vi "73XX Motion Controller RT Driver VI.vi"(7 "Operation":T1, 11 "Device Reference in":T2 format="%.0x") -> (0 "Error Code":i32)   [LabVIEW 2010, in "73XX Motion Controller Custom Device.lvlib"]
uses:
  73XX Motion Controller Custom Device.lvlib
  <vilib>/NI VeriStand/Custom Device API/Custom Device Item Ref.ctl
  <vilib>/NI VeriStand/Custom Device API/Hardware Interface Driver VI Operation.ctl
  <vilib>/NI VeriStand/Custom Device API/Data Reference.ctl
  <vilib>/NI VeriStand/Custom Device API/Custom Device Channel Type.ctl
  <vilib>/NI VeriStand/Custom Device API/Data Access Type.ctl
  <vilib>/NI VeriStand/Custom Device API/Get Item Property (U16).vi
  <vilib>/Motion/FlexMotion/FunctionsVIs/StartStopMotion.llb/Start Motion (8 axes).flx
  <vilib>/Motion/FlexMotion/FunctionsVIs/StartStopMotion.llb/Stop Motion (8 axes).flx
  <vilib>/NI Veristand/Custom Device API/Custom Device API.lvlib
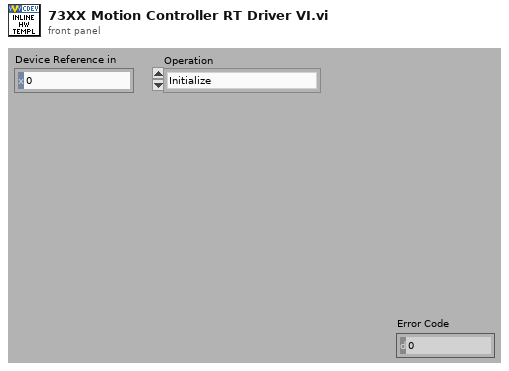
[diagram p1: front panel]
types:
  T1 = typedef "Custom Device API.lvlib/Hardware Interface Driver VI Operation.ctl" = enum16{"Initialize", "Start", "Read Data from HW", "Write Data to HW", "Close"}
  T2 = typedef "Custom Device API.lvlib/Custom Device Item Ref.ctl" = u64
  T3 = typedef "Custom Device API.lvlib/Data Reference.ctl" = i32
  T4 = cluster{"Device Error":errorcluster, "Current Position":i32, "Board ID":u16, "Axis":u16, "Velocity":u16, "Velocity Ref":T3, "Current Position Ref":T3, "Current Velcoity":i32, "Target Position":i32, "Target Position Ref":T3, "Current Velocity Ref":T3, "Reset Position? Ref":T3, "Reset Position?":T3, "Operation Mode":T3}
  T5 = typedef "Custom Device API.lvlib/Custom Device Channel Type.ctl" = enum16{"Input", "Output"}
  T6 = enum16{"Absolute Position", "Relative Position", "Velocity", "Relative to Cap Pos", "Modulus Position", "Absolute Contouring", "Relative Contouring"}
  T7 = typedef "Custom Device API.lvlib/Data Access Type.ctl" = enum16{"Read", "Write"}
  T8 = typedef "Bd Id Out" = u8
  T9 = typedef "Resource Out (Enum).flx" = u16
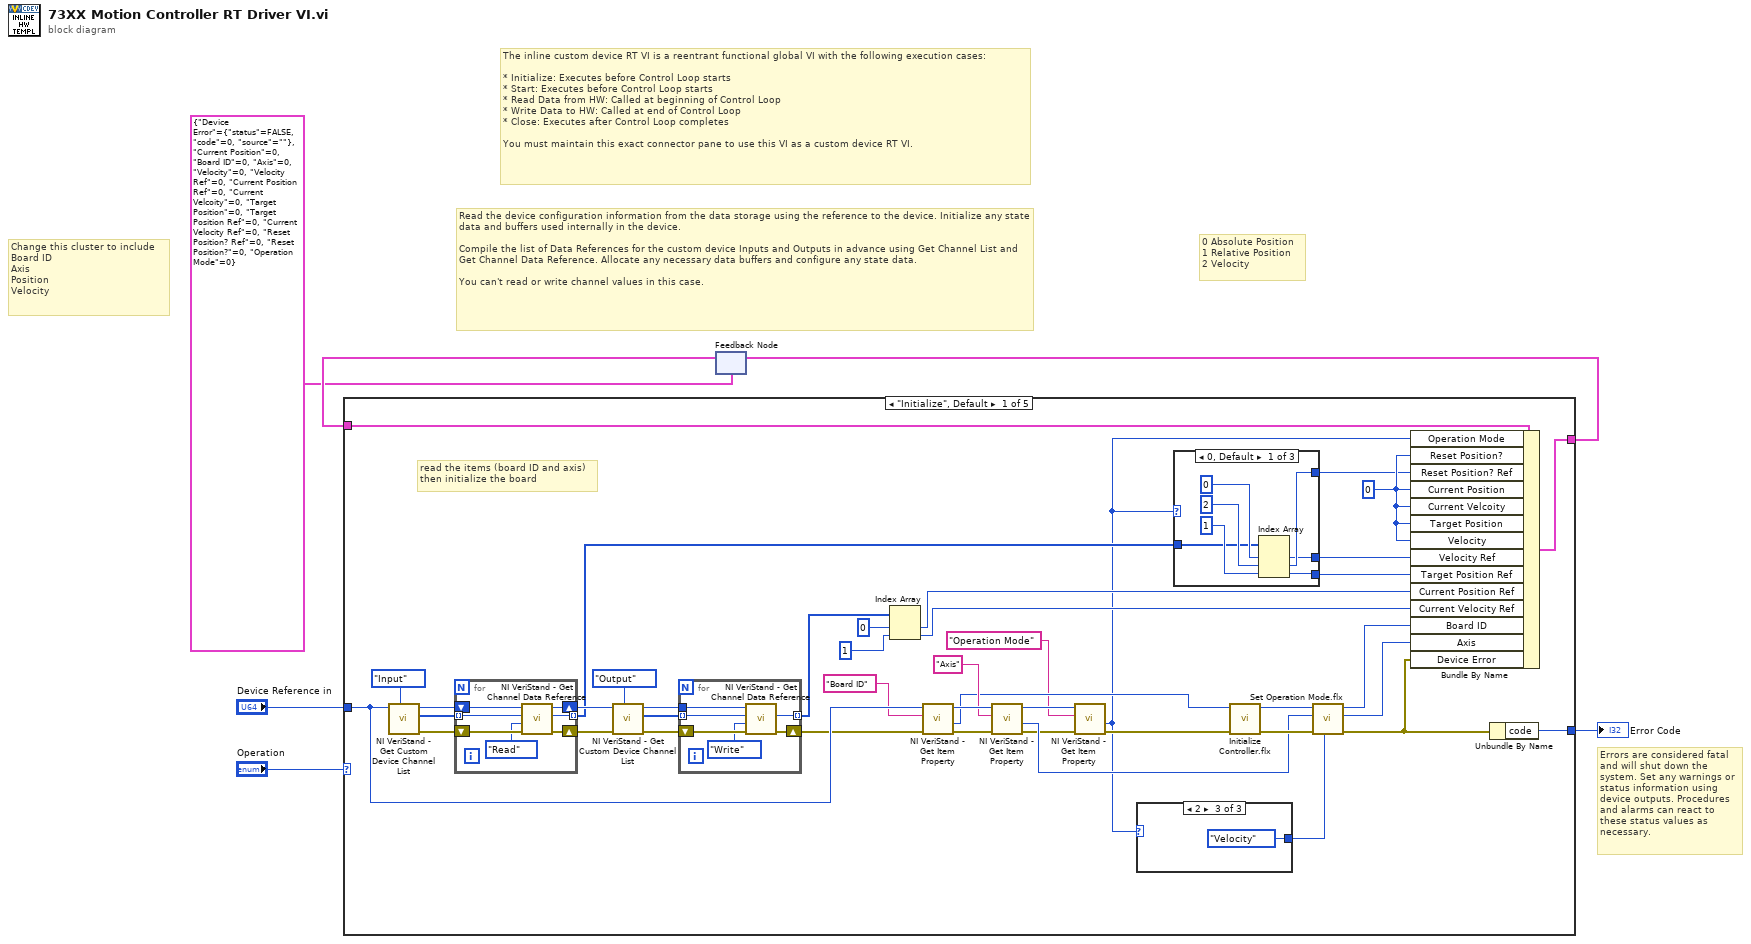
[diagram p0: block diagram]
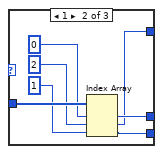
[diagram p2: hidden frame]
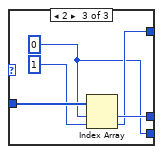
[diagram p3: hidden frame]
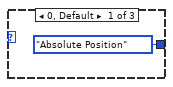
[diagram p4: hidden frame]
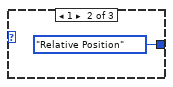
[diagram p5: hidden frame]
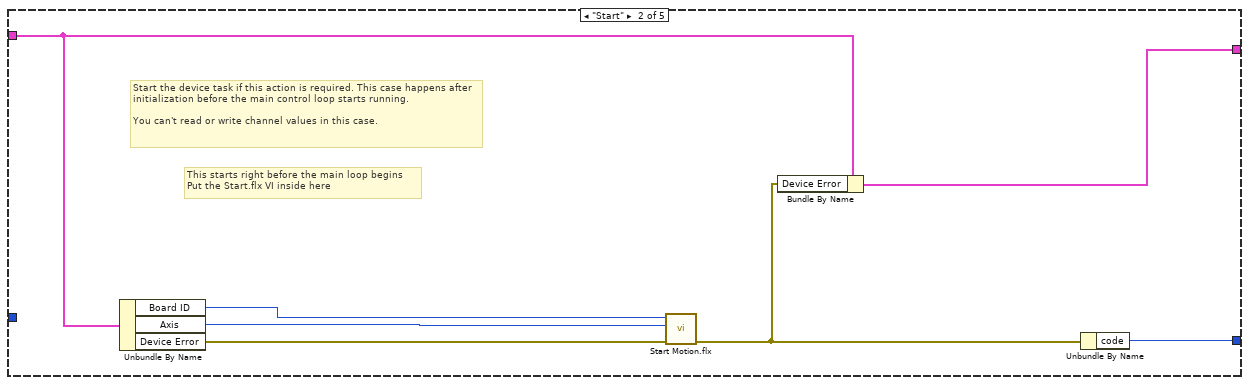
[diagram p6: hidden frame]
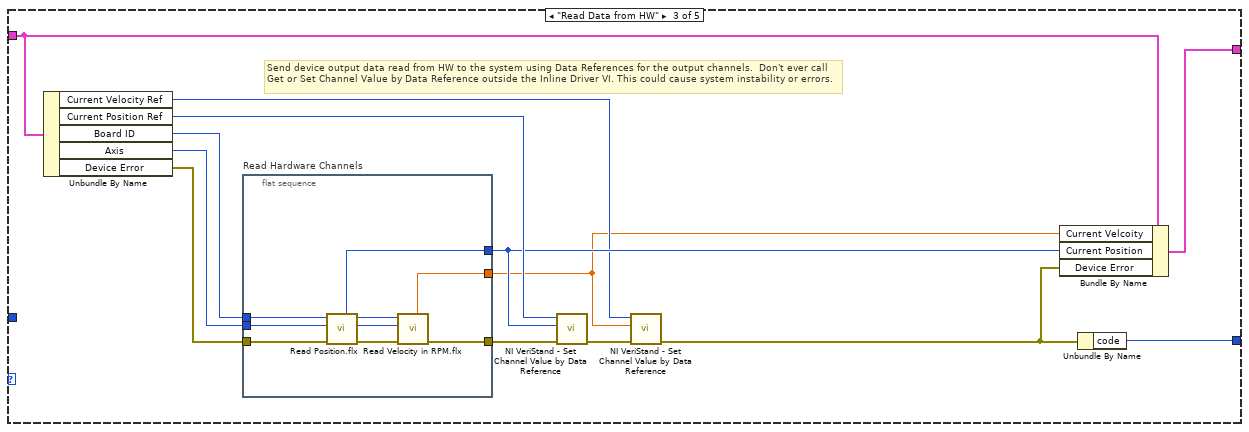
[diagram p7: hidden frame]
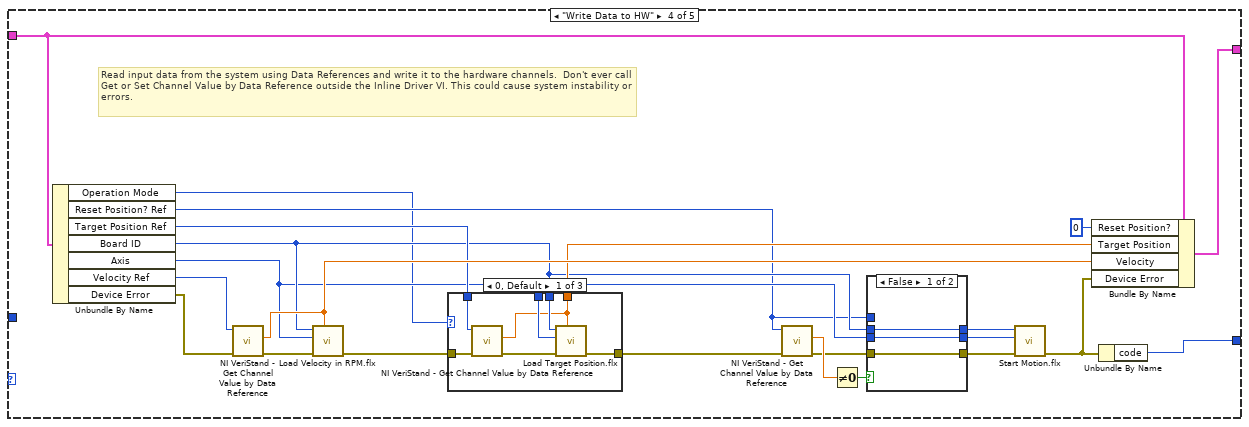
[diagram p8: hidden frame]
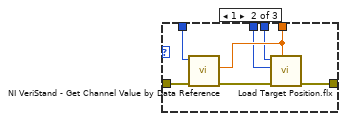
[diagram p9: hidden frame]
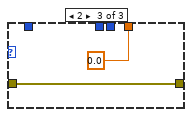
[diagram p10: hidden frame]
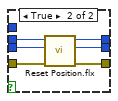
[diagram p11: hidden frame]
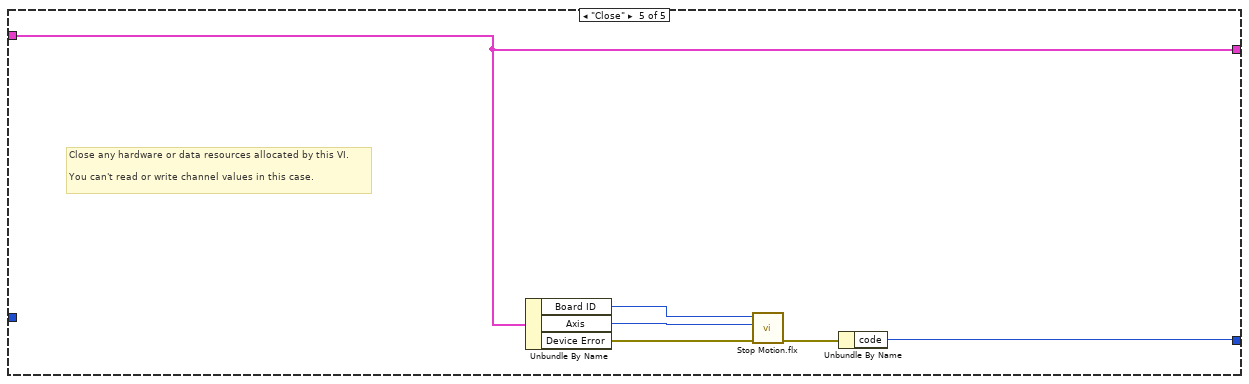
[diagram p12: hidden frame]
diagram:
  # "0 Absolute Position\n1 Relative Position\n2 Velocity"
  # "Change this cluster to include\nBoard ID\nAxis\nPosition\nVelocity"
  # "Read the device configuration information from the data storage using the reference to the device. Initialize any state data and buffers used internally in the device.\n\nCompile the list of Data References for the custom device Inputs and Outputs in advance using Get Channel List and Get Channel Data Reference. Allocate any necessary data buffers and configure any state data.\n\nYou can't read or write channel values in this case."
  # "Errors are considered fatal and will shut down the system. Set any warnings or status information using device outputs. Procedures and alarms can react to these status values as necessary."
  # "The inline custom device RT VI is a reentrant functional global VI with the following execution cases:\n\n* Initialize: Executes before Control Loop starts\n* Start: Executes before Control Loop starts\n* Read Data from HW: Called at beginning of Control Loop\n* Write Data to HW: Called at end of Control Loop\n* Close: Executes after Control Loop completes\n\nYou must maintain this exact connector pane to use this VI as a custom device RT VI."
  n1 = feedback #1(T4 {"Device Error"={"status"=FALSE, "code"=0, "source"=""}, "Current Position"=0, "Board ID"=0, "Axis"=0, "Velocity"=0, "Velocity Ref"=0, "Current Position Ref"=0, "Current Velcoity"=0, "Target Position"=0, "Target Position Ref"=0, "Current Velocity Ref"=0, "Reset Position? Ref"=0, "Reset Position?"=0, "Operation Mode"=0} ("cluster")) -> (w4:T4)
  n2 = case shown="\"Initialize\", Default" "Operation" {
    tunnel: [w27 w89 w99 w134 w166] -> w5
    tunnel: w4 -> [w28 w90 w100 w135 w166]
    tunnel: "Device Reference in" -> [w35 _ _ _ _]
    tunnel: [w47 w87 w102 w132 w161] -> w2
    frame "Initialize", Default {
      w14 = 0 ("element")
      # "read the items (board ID and axis)\nthen initialize the board"
      n3 = call <vilib>:"NI VeriStand - Get Custom Device Channel List.vi"("Channel Type"=Custom_Device_Channel_Type."Input", "Device Ref in"=w35) -> ("error out"=w45:errorcluster, "Specified Channel Ref List"=w44:T2[], "Device Ref out"=w46:T2)  [unwired: 1 in, 6 out]
      n4 = for {
        shift-right: [w78] -> w40
        shift-left: w46 -> [w82]
        tunnel: w44 -> [w81] mode=indexing
        shift-right: [w79] -> w39
        shift-left: w45 -> [w83]
        tunnel: [w77] -> w30 mode=indexing
        n5 = call <vilib>:"NI VeriStand - Get Channel Data Reference.vi"("error in (no error)"=w83, "Access"=Data_Access_Type."Read", "Channel Ref in"=w81, "Device Ref in"=w82) -> ("error out"=w79:errorcluster, "Channel Data Reference"=w77:T3, "Device Ref out"=w78:T2)  [unwired: 5 out]
      }
      n6 = call <vilib>:"NI VeriStand - Get Custom Device Channel List.vi"("Channel Type"=Custom_Device_Channel_Type."Output", "error in (no error)"=w39, "Device Ref in"=w40) -> ("error out"=w43:errorcluster, "Specified Channel Ref List"=w38:T2[], "Device Ref out"=w42:T2)  [unwired: 6 out]
      n7 = for {
        tunnel: w38 -> [w74] mode=indexing
        shift-right: [w72] -> w32
        shift-left: w43 -> [w76]
        tunnel: [w71] -> w31 mode=indexing
        tunnel: w42 -> [w75]
        n8 = call <vilib>:"NI VeriStand - Get Channel Data Reference.vi"("error in (no error)"=w76, "Access"=Data_Access_Type."Write", "Channel Ref in"=w74, "Device Ref in"=w75) -> ("error out"=w72:errorcluster, "Channel Data Reference"=w71:T3)  [unwired: 6 out]
      }
      n9 = Index Array(array=w31, index #1=0 ("index"), index #2=1 ("index")) -> (element #1=w25:T3, element #2=w23:T3)
      n10 = call-poly <vilib>:"NI VeriStand - Get Item Property.vi"("error in (no error)"=w32, "Property Name"="Board ID", "Item Ref in"=w35) -> ("error out"=w36:errorcluster, "Value"=w22:u16, "Item Ref out"=w37:T2)  [unwired: 5 in, 1 out]
      n11 = call-poly <vilib>:"NI VeriStand - Get Item Property.vi"("error in (no error)"=w36, "Property Name"="Axis", "Item Ref in"=w37) -> ("error out"=w13:errorcluster, "Value"=w19:u16, "Item Ref out"=w11:T2)  [unwired: 5 in, 1 out]
      n12 = call-poly <vilib>:"NI VeriStand - Get Item Property.vi"("error in (no error)"=w13, "Property Name"="Operation Mode", "Item Ref in"=w11) -> ("error out"=w12:errorcluster, "Value"=w7:u16)  [unwired: 5 in, 2 out]
      n13 = case shown="2" w7 {
        tunnel: [T6."Absolute Position" ("Position Mode (Absolute)") T6."Relative Position" ("Position Mode (Absolute)") T6."Velocity" ("Position Mode (Absolute)")] -> w18
        frame 0, Default {
        }
        frame 1 {
        }
        frame 2 {
        }
      }
      n14 = case shown="0, Default" w7 {
        tunnel: w30 -> [w51 w62 w67]
        tunnel: [w50 w60 w66] -> w26
        tunnel: [w49 w57 w63] -> w9
        tunnel: [w52 w56 w64] -> w8
        frame 0, Default {
          n15 = Index Array(array=w51, index #1=0 ("index"), index #2=2 ("index"), index #3=1 ("index")) -> (element #1=w50:T3, element #2=w52:T3, element #3=w49:T3)
        }
        frame 1 {
          n16 = Index Array(array=w62, index #1=0 ("index"), index #2=2 ("index"), index #3=1 ("index")) -> (element #1=w60:T3, element #2=w56:T3, element #3=w57:T3)
        }
        frame 2 {
          w63 = 0 ("index")
          n17 = Index Array(array=w67, index #1=w63, index #2=1 ("index")) -> (element #1=w66:T3, element #2=w64:T3)
        }
      }
      n18 = call <vilib>:"Initialize Controller.flx"("error in (no error)"=w12, "Board ID"=w22) -> ("error out"=w21:errorcluster, "Bd ID Out"=w20:T8)  [unwired: 6 in]
      n19 = call <vilib>:"Set Operation Mode.flx"("Position Mode (Absolute)"=w18, "error in (no error)"=w21, "Axis or Vector Space"=w19, "Board ID"=w20) -> ("error out"=w17:errorcluster, "Resource Output"=w15:T9, "Bd ID Out"=w16:T8)  [unwired: 2 in]
      n20 = Bundle By Name(cluster=w28, "Operation Mode"=w7, "Reset Position?"=w14, "Reset Position? Ref"=w8, "Current Position"=w14, "Current Velcoity"=w14, "Target Position"=w14, "Velocity"=w14, "Velocity Ref"=w26, "Target Position Ref"=w9, "Current Position Ref"=w25, "Current Velocity Ref"=w23, "Board ID"=w16, "Axis"=w15, "Device Error"=w17) -> (w27:T4)
      n21 = Unbundle By Name(w17) -> ("code"=w47:i32)
    }
    frame "Start" {
      # "This starts right before the main loop begins\nPut the Start.flx VI inside here"
      # "Start the device task if this action is required. This case happens after initialization before the main control loop starts running.\n\nYou can't read or write channel values in this case."
      n22 = Unbundle By Name(w90) -> ("Board ID"=w86:u16, "Axis"=w84:u16, "Device Error"=w85:errorcluster)
      n23 = call-poly <vilib>:"Start Motion.flx"("error in (no error)"=w85, "Axis or Vector Space"=w84, "Board ID"=w86) -> ("error out"=w88:errorcluster)  [unwired: 3 in, 2 out]
      n24 = Bundle By Name(cluster=w90, "Device Error"=w88) -> (w89:T4)
      n25 = Unbundle By Name(w88) -> ("code"=w87:i32)
    }
    frame "Read Data from HW" {
      # "Send device output data read from HW to the system using Data References for the output channels.  Don't ever call Get or Set Channel Value by Data Reference outside the Inline Driver VI. This could cause system instability or errors."
      n26 = Unbundle By Name(w100) -> ("Current Velocity Ref"=w92:T3, "Current Position Ref"=w96:T3, "Board ID"=w97:u16, "Axis"=w101:u16, "Device Error"=w98:errorcluster)
      n27 = flat-sequence "Read Hardware Channels" {
        tunnel: w98 -> [w112]
        tunnel: [w107] -> w103
        tunnel: w101 -> [w111]
        tunnel: w97 -> [w110]
        tunnel: [w109] -> w95
        tunnel: [w104] -> w91
        frame #0 {
          n28 = call <vilib>:"Read Position.flx"("error in (no error)"=w112, "Axis"=w111, "Board ID"=w110) -> ("error out"=w108:errorcluster, "Resource Output"=w105:T9, "Bd ID Out"=w106:T8, "Position"=w109:i32)  [unwired: 3 in]
          n29 = call <vilib>:"Read Velocity in RPM.flx"("error in (no error)"=w108, "Axis or Vector Space"=w105, "Board ID"=w106) -> ("error out"=w107:errorcluster, "Filtered Velocity"=w104:dbl)  [unwired: 3 in, 2 out]
        }
      }
      n30 = call <vilib>:"NI VeriStand - Set Channel Value by Data Reference.vi"("error in (no error)"=w103, "Value"=w95, "Data Reference in"=w96) -> ("error out"=w94:errorcluster)  [unwired: 8 out]
      n31 = call <vilib>:"NI VeriStand - Set Channel Value by Data Reference.vi"("error in (no error)"=w94, "Value"=w91, "Data Reference in"=w92) -> ("error out"=w93:errorcluster)  [unwired: 8 out]
      n32 = Bundle By Name(cluster=w100, "Current Velcoity"=w91, "Current Position"=w95, "Device Error"=w93) -> (w99:T4)
      n33 = Unbundle By Name(w93) -> ("code"=w102:i32)
    }
    frame "Write Data to HW" {
      # "Read input data from the system using Data References and write it to the hardware channels.  Don't ever call Get or Set Channel Value by Data Reference outside the Inline Driver VI. This could cause system instability or errors."
      n34 = Unbundle By Name(w135) -> ("Operation Mode"=w113:T3, "Reset Position? Ref"=w114:T3, "Target Position Ref"=w126:T3, "Board ID"=w117:u16, "Axis"=w116:u16, "Velocity Ref"=w129:T3, "Device Error"=w131:errorcluster)
      n35 = call <vilib>:"NI VeriStand - Get Channel Value by Data Reference.vi"("error in (no error)"=w131, "Data Reference in"=w129) -> ("error out"=w133:errorcluster, "Value"=w128:dbl)  [unwired: 8 out]
      n36 = call <vilib>:"Load Velocity in RPM.flx"("Velocity (500)"=w128, "error in (no error)"=w133, "Axis or Vector Space"=w116, "Board ID"=w117) -> ("error out"=w127:errorcluster)  [unwired: 3 in, 2 out]
      n37 = case shown="0, Default" w113 {
        tunnel: w127 -> [w140 w149 w151]
        tunnel: w126 -> [w139 w148 _]
        tunnel: [w136 w146 0.0 ("Value")] -> w125
        tunnel: [w141 w145 w151] -> w121
        tunnel: w117 -> [w138 w144 _]
        tunnel: w116 -> [w137 w143 _]
        frame 0, Default {
          n38 = call <vilib>:"NI VeriStand - Get Channel Value by Data Reference.vi"("error in (no error)"=w140, "Data Reference in"=w139) -> ("error out"=w142:errorcluster, "Value"=w136:dbl)  [unwired: 8 out]
          n39 = call <vilib>:"Load Target Position.flx"("Target Position (0)"=w136, "error in (no error)"=w142, "Axis"=w137, "Board ID"=w138) -> ("error out"=w141:errorcluster)  [unwired: 3 in, 2 out]
        }
        frame 1 {
          n40 = call <vilib>:"NI VeriStand - Get Channel Value by Data Reference.vi"("error in (no error)"=w149, "Data Reference in"=w148) -> ("error out"=w147:errorcluster, "Value"=w146:dbl)  [unwired: 8 out]
          n41 = call <vilib>:"Load Target Position.flx"("Target Position (0)"=w146, "error in (no error)"=w147, "Axis"=w143, "Board ID"=w144) -> ("error out"=w145:errorcluster)  [unwired: 3 in, 2 out]
        }
        frame 2 {
        }
      }
      n42 = call <vilib>:"NI VeriStand - Get Channel Value by Data Reference.vi"("error in (no error)"=w121, "Data Reference in"=w114) -> ("error out"=w118:errorcluster, "Value"=w120:dbl)  [unwired: 8 out]
      n43 = Not Equal To 0?(x=w120) -> (x != 0?=w119:bool)
      n44 = case shown="False" w119 {
        tunnel: w118 -> [w154 w160]
        tunnel: [w154 w155] -> w124
        tunnel: [w152 w156] -> w123
        tunnel: [w153 w157] -> w122
        tunnel: w117 -> [w153 w159]
        tunnel: w116 -> [w152 w158]
        tunnel: w114 -> [_ _]
        frame False {
        }
        frame True {
          n45 = call <vilib>:"Reset Position.flx"("error in (no error)"=w160, "Axis"=w158, "Board ID"=w159) -> ("error out"=w155:errorcluster, "Resource Output"=w156:T9, "Bd ID Out"=w157:T8)  [unwired: 4 in]
        }
      }
      n46 = call-poly <vilib>:"Start Motion.flx"("error in (no error)"=w124, "Axis or Vector Space"=w123, "Board ID"=w122) -> ("error out"=w130:errorcluster)  [unwired: 3 in, 2 out]
      n47 = Bundle By Name(cluster=w135, "Reset Position?"=T3 0, "Target Position"=w125, "Velocity"=w128, "Device Error"=w130) -> (w134:T4)
      n48 = Unbundle By Name(w130) -> ("code"=w132:i32)
    }
    frame "Close" {
      # "Close any hardware or data resources allocated by this VI.\n\nYou can't read or write channel values in this case."
      n49 = Unbundle By Name(w166) -> ("Board ID"=w165:u16, "Axis"=w164:u16, "Device Error"=w163:errorcluster)
      n50 = call-poly <vilib>:"Stop Motion.flx"("error in (no error)"=w163, "Axis or Vector Space"=w164, "Board ID"=w165) -> ("error out"=w162:errorcluster)  [unwired: 4 in, 2 out]
      n51 = Unbundle By Name(w162) -> ("code"=w161:i32)
    }
  }
  "Error Code" <- w2
  n52 = feedback-in #1(w5) -> ()
